vi "GainToCtrlV.vi"(8 "error in (no error)":errorcluster, 10 "Gain":dbl, 11 "Channel":enum16{"Ch1", "Ch2", "Ch3", "Ch4"}(ring)) -> (0 "error out":errorcluster, 3 "CtrlV":dbl)   [LabVIEW 2020]
uses:
  APD/APDClass.lvclass
  <vilib>/gmath/NI_Gmath.lvlib
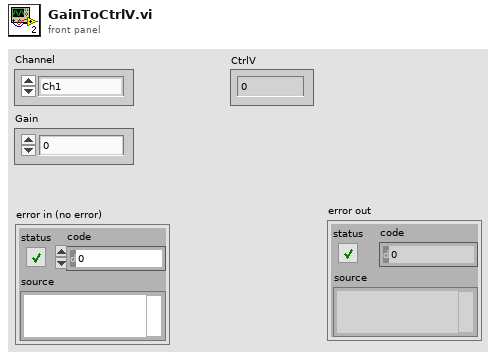
[diagram p1: front panel]
types:
  T1 = typedef "GainData.ctl" = cluster{"CtrlV":dbl[], "NumOfWFs":i32, "WF length":i32, "Gain":dbl[], "GainRaw":dbl[][], "GainBGRaw":dbl[][]}
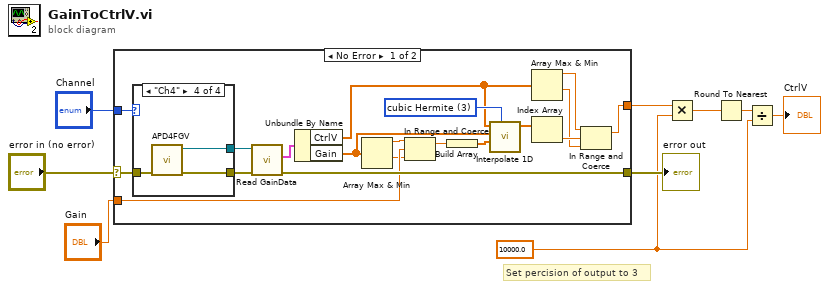
[diagram p0: block diagram]
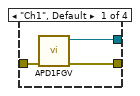
[diagram p2: hidden frame]
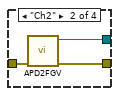
[diagram p3: hidden frame]
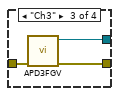
[diagram p4: hidden frame]
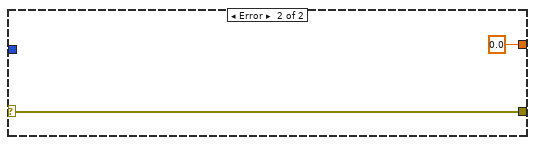
[diagram p5: hidden frame]
diagram:
  w2 = 10000.0 ("y")
  # "Set percision of output to 3"
  n1 = case shown="No Error" "error in (no error)" {
    selector: "error in (no error)" -> [w20 w41]
    tunnel: "Channel" -> [w28 _]
    tunnel: "Gain" -> [w13 _]
    tunnel: [w18 0.0 ("Numeric")] -> w5
    tunnel: [w21 w41] -> w7
    frame No Error {
      w23 = 3 items=["nearest", "linear", "spline", "cubic Hermite", "Lagrange"] ("method")
      n2 = case shown="\"Ch4\"" w28 {
        tunnel: [w31 w33 w36 w39] -> w27
        tunnel: [w30 w34 w37 w40] -> w26
        tunnel: w20 -> [w29 w32 w35 w38]
        frame "Ch1", Default {
          n3 = call "APD1FGV.vi"("Error In"=w29) -> ("Error Out"=w31:errorcluster, "APDClass out"=w30:refnum<class "APDClass.lvclass">)  [unwired: 9 in]
        }
        frame "Ch2" {
          n4 = call "APD2FGV.vi"("Error In"=w32) -> ("Error Out"=w33:errorcluster, "APDClass out"=w34:refnum<class "APDClass.lvclass">)  [unwired: 9 in]
        }
        frame "Ch3" {
          n5 = call "APD3FGV.vi"("Error In"=w35) -> ("Error Out"=w36:errorcluster, "APDClass out"=w37:refnum<class "APDClass.lvclass">)  [unwired: 9 in]
        }
        frame "Ch4" {
          n6 = call "APD4FGV.vi"("Error In"=w38) -> ("Error Out"=w39:errorcluster, "APDClass out"=w40:refnum<class "APDClass.lvclass">)  [unwired: 9 in]
        }
      }
      n7 = call-dynamic "Read GainData.vi"("error in (no error)"=w27, "APDClass in"=w26) -> ("error out"=w21:errorcluster, "GainData"=w25:T1)  [unwired: 7 in, 1 out]
      n8 = Unbundle By Name(w25) -> ("CtrlV"=w17:dbl[], "Gain"=w14:dbl[])
      n9 = Array Max & Min(array=w14) -> (max value=w12:dbl, min value=w11:dbl)  [unwired: 2 out]
      n10 = In Range and Coerce(upper limit=w12, x=w13, lower limit=w11) -> (coerced(x)=w10:dbl)  [unwired: 1 out]
      n11 = Build Array(w10) -> (w24:dbl[])
      n12 = call <vilib>:"Interpolate 1D.vi"("method"=w23, "xi"=w24, "X"=w14, "Y"=w17) -> ("yi"=w22:dbl[])  [unwired: 5 in, 2 out]
      n13 = Array Max & Min(array=w17) -> (max value=w16:dbl, min value=w15:dbl)  [unwired: 2 out]
      n14 = Index Array(array=w22) -> (element=w19:dbl)  [unwired: 1 in]
      n15 = In Range and Coerce(upper limit=w16, x=w19, lower limit=w15) -> (coerced(x)=w18:dbl)  [unwired: 1 out]
    }
    frame Error {
    }
  }
  "error out" <- w7
  n16 = Multiply(x=w5, y=w2) -> (x*y=w4:dbl)
  n17 = Round To Nearest(number=w4) -> (nearest integer value=w3:dbl)
  n18 = Divide(x=w3, y=w2) -> (x/y=→"CtrlV":dbl)
